vi "Load Programs.vi"(0 "Program List in":refnum<class "Program List.lvclass">, 5 "error in (no error)":errorcluster, 8 "Application.lvclass":refnum<class "Application.lvclass">) -> (14 "Program List out":refnum<class "Program List.lvclass">, 15 "Programs":string[](array[string]), 19 "error out":errorcluster)   [LabVIEW 2019, in "Program List.lvclass"]
uses:
  Program List.lvclass
  Application.lvclass
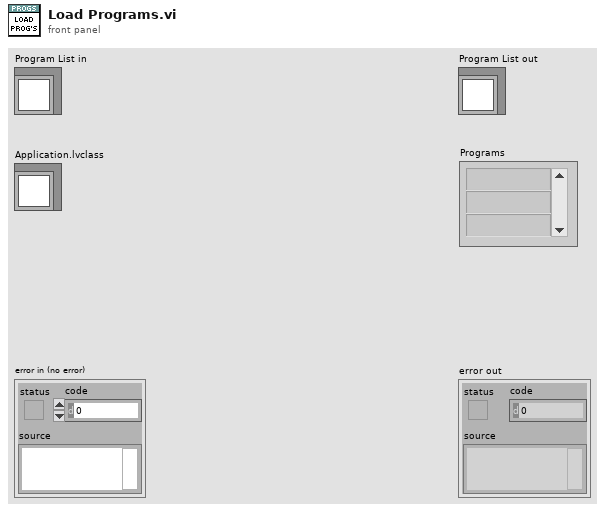
[diagram p1: front panel]
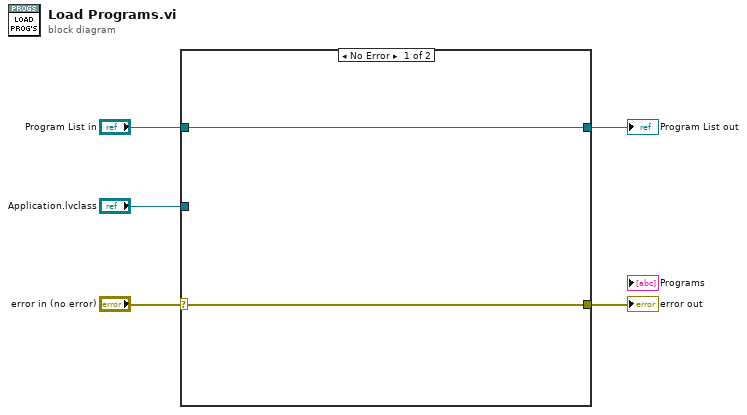
[diagram p0: block diagram]
diagram:
  n1 = case shown="No Error" "error in (no error)" {
    selector: "error in (no error)" -> [w6 w9]
    tunnel: [w6 w9] -> w4
    tunnel: [w7 w8] -> w2
    tunnel: "Program List in" -> [w7 w8]
    tunnel: "Application.lvclass" -> [_ _]
    frame No Error {
    }
    frame Error {
    }
  }
  "error out" <- w4
  "Program List out" <- w2
